vi "Page_Advanced_WriteAll.vi"(6 "ctl references":T1, 8 "error in (no error)":errorcluster, 11 "AB_DLL in":refnum<class "AB_DLL.lvclass">) -> (0 "error out":errorcluster, 3 "AB_DLL out":refnum<class "AB_DLL.lvclass">)   [LabVIEW 2020, in "AB_DLL.lvclass"]
uses:
  <vilib>/AppBuilder/AB_Classes/DLL/AB_DLL.lvclass
  e:/builds/penguin/labview/branches/2020/dev/dist/vi.lib/AppBuilder/AB_Classes/TargetFile/AB_Targetfile.lvclass
  <resource>/Framework/Providers/Builds/AppBuilder/AB_UI_Page_Advanced_References.ctl
  <vilib>/AppBuilder/AB_Classes/DLL/AB_DLL.lvclass/AB_DLL.ctl
  <vilib>/AppBuilder/AB_Classes/Application/AB_Application.lvclass
  <vilib>/AppBuilder/AB_Classes/TargetFile/AB_Targetfile.lvclass
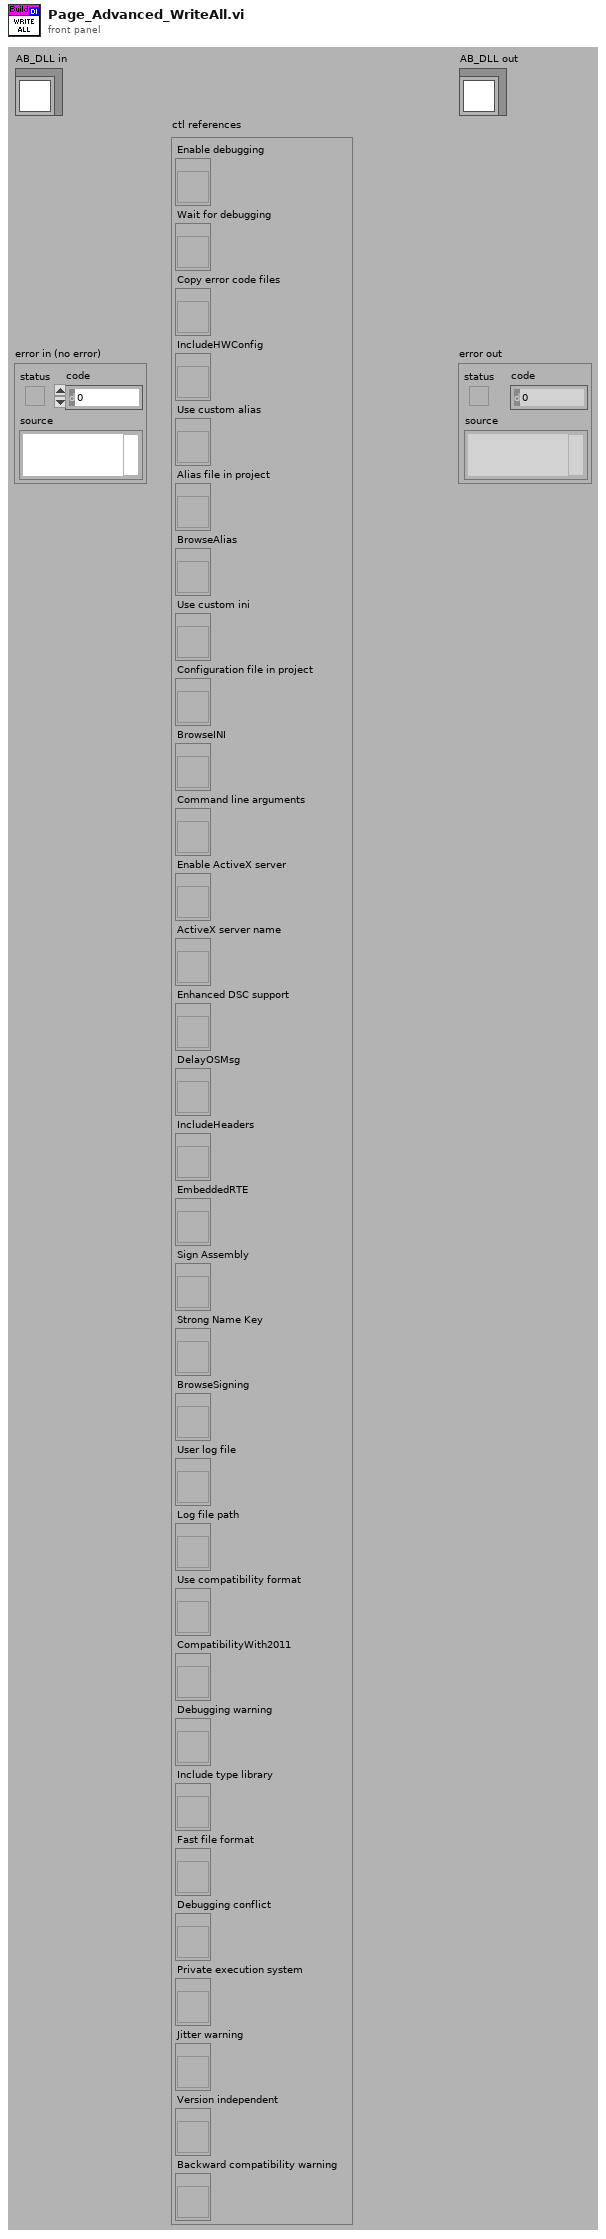
[diagram p1: front panel]
types:
  T1 = typedef "AB_UI_Page_Advanced_References.ctl" = cluster{"Enable debugging":refnum<vi>, "Wait for debugging":refnum<vi>, "Copy error code files":refnum<vi>, "IncludeHWConfig":refnum<vi>, "Use custom alias":refnum<vi>, "Alias file in project":refnum<vi>, "BrowseAlias":refnum<vi>, "Use custom ini":refnum<vi>, "Configuration file in project":refnum<vi>, "BrowseINI":refnum<vi>, "Command line arguments":refnum<vi>, "Enable ActiveX server":refnum<vi>, "ActiveX server name":refnum<vi>, "Enhanced DSC support":refnum<vi>, "DelayOSMsg":refnum<vi>, "IncludeHeaders":refnum<vi>, "EmbeddedRTE":refnum<vi>, "Sign Assembly":refnum<vi>, "Strong Name Key":refnum<vi>, "BrowseSigning":refnum<vi>, "User log file":refnum<vi>, "Log file path":refnum<vi>, "Use compatibility format":refnum<vi>, "CompatibilityWith2011":refnum<vi>, "Debugging warning":refnum<vi>, "Include type library":refnum<vi>, "Fast file format":refnum<vi>, "Debugging conflict":refnum<vi>, "Private execution system":refnum<vi>, "Jitter warning":refnum<vi>, "Version independent":refnum<vi>, "Backward compatibility warning":refnum<vi>}
  T2 = typedef "AB_Targetfile.ctl" = cluster{"targetfileName":string, "targetfileGUID":string, "enableDebugging":bool, "versionInfo":cluster{"productName":string, "legalCopyright":string, "companyName":string, "internalName":string, "fileDescription":string}, "eng_consolidatedTypeInfo":string, "fastFileFormat":bool, "eng_LEIFBuildData":u32, "versionIndependent":bool}
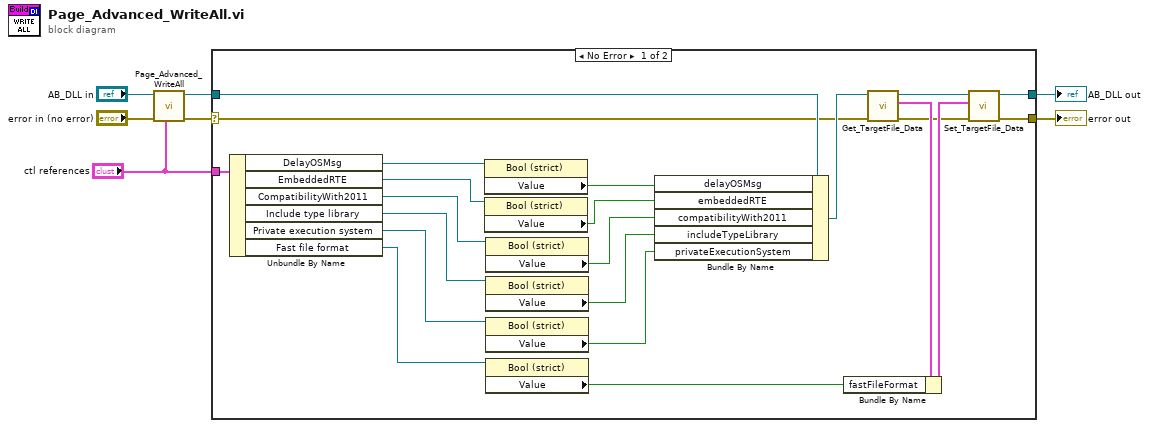
[diagram p0: block diagram]
diagram:
  n1 = call-parent "Page_Advanced_WriteAll.vi"("ctl references"="ctl references", "error in (no error)"="error in (no error)", "AB_Application in"="AB_DLL in") -> ("error out"=w5:errorcluster, "AB_Application out"=w4:refnum<class "AB_DLL.lvclass">)  [unwired: 7 in]
  n2 = case shown="No Error" w5 {
    selector: w5 -> [w13 w30]
    tunnel: w4 -> [w29 w31]
    tunnel: [w14 w31] -> w3
    tunnel: [w11 w30] -> w2
    tunnel: "ctl references" -> [w28 _]
    frame No Error {
      n3 = Unbundle By Name(w28) -> ("DelayOSMsg"=w27:refnum<vi>, "EmbeddedRTE"=w25:refnum<vi>, "CompatibilityWith2011"=w23:refnum<vi>, "Include type library"=w21:refnum<vi>, "Private execution system"=w9:refnum<vi>, "Fast file format"=w10:refnum<vi>)
      n4 = property class="Bool (strict)"(reference=w27) -> ("Value"=w26:bool)  [unwired: 1 in, 2 out]
      n5 = property class="Bool (strict)"(reference=w25) -> ("Value"=w24:bool)  [unwired: 1 in, 2 out]
      n6 = property class="Bool (strict)"(reference=w23) -> ("Value"=w22:bool)  [unwired: 1 in, 2 out]
      n7 = property class="Bool (strict)"(reference=w21) -> ("Value"=w20:bool)  [unwired: 1 in, 2 out]
      n8 = property class="Bool (strict)"(reference=w9) -> ("Value"=w8:bool)  [unwired: 1 in, 2 out]
      n9 = property class="Bool (strict)"(reference=w10) -> ("Value"=w16:bool)  [unwired: 1 in, 2 out]
      n10 = Bundle By Name(cluster=w29, "delayOSMsg"=w26, "embeddedRTE"=w24, "compatibilityWith2011"=w22, "includeTypeLibrary"=w20, "privateExecutionSystem"=w8) -> (w15:refnum<class "AB_DLL.lvclass">)
      n11 = call <vilib>:"Get_TargetFile_Data.vi"("error in (no error)"=w13, "AB_Targetfile in"=w15) -> ("error out"=w12:errorcluster, "data"=w18:T2, "AB_Targetfile out"=w19:refnum<class "AB_DLL.lvclass">)  [unwired: 7 in]
      n12 = Bundle By Name(cluster=w18, "fastFileFormat"=w16) -> (w17:T2)
      n13 = call <vilib>:"Set_TargetFile_Data.vi"("error in (no error)"=w12, "data"=w17, "AB_Targetfile in"=w19) -> ("error out"=w11:errorcluster, "AB_Targetfile out"=w14:refnum<class "AB_DLL.lvclass">)  [unwired: 7 in]
    }
    frame Error {
    }
  }
  "error out" <- w2
  "AB_DLL out" <- w3
